vi "Begin.vi"(8 "error in":errorcluster) -> (0 "error out":errorcluster)   [LabVIEW 2018]
doc: "Called before other user functions, this VI is expected to open initial I/O refnums, load in file data, and do all program initialization. Notice that the <B>error out</B> terminal is simply used for data flow. Wiring it to other structures or subVIs ensures that this VI runs first."
uses:
  <vilib>/Rock Robotics/WPI/DriverStation/WPI_DriverStationRobotMode2.ctl
  <vilib>/Rock Robotics/WPI/Joystick/WPI_JoystickDeviceEnum.ctl
  <vilib>/Rock Robotics/SystemInterfaces/AI/FPGA_AIChannel.ctl
  <vilib>/Rock Robotics/WPI/Solenoid/WPI_SolenoidChannel.ctl
  <vilib>/Rock Robotics/SystemInterfaces/DIO/FPGA_DIORelayChannel.ctl
  <vilib>/Rock Robotics/WPI/Relay/WPI_RelayValue.ctl
  <vilib>/Rock Robotics/SystemInterfaces/DIO/FPGA_DIOPWMChannel.ctl
  <vilib>/Rock Robotics/SystemInterfaces/spilib/spi_bus.ctl
  <vilib>/Rock Robotics/SystemInterfaces/DIO/FPGA_DIOChannel.ctl
  Robot Global Data.vi
  <vilib>/Rock Robotics/WPI/Solenoid/WPI_SolenoidOpenSingle.vi
  <vilib>/Rock Robotics/WPI/Utilities/WPI_GetSetVariantRefNum.vi
  <vilib>/Rock Robotics/WPI/MotorControl/WPI_MotorControlOpen VictorSP.vi
  navx-mxp/labview/navX Library v2/IO/Open/Z900_navX_Open_SPI.vi
  <vilib>/Rock Robotics/WPI/Counter/WPI_CounterDigitalInputToDigitalSource.vi
  navx-mxp/labview/navX Library v2/navX Library v2.lvlib
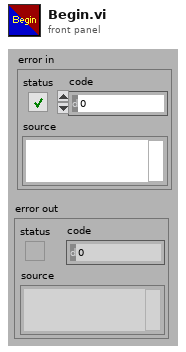
[diagram p1: front panel]
types:
  T1 = typedef "WPI_DriverStationRobotMode2.ctl" = enum16{"Autonomous Disabled", "Autonomous Enabled", "Teleop Disabled", "Teleop Enabled", "Disconnected", "Finish", "Test Disabled", "Test Enabled", "Emergency Stopped"}
  T2 = typedef "WPI_JoystickDeviceEnum.ctl" = enum16{"USB 0", "USB 1", "USB 2", "USB 3", "USB 4", "USB 5"}
  T3 = typedef "FPGA_AIChannel.ctl" = enum8{"AI 0", "AI 1", "AI 2", "AI 3", "AI MXP 0", "AI MXP 1", "AI MXP 2", "AI MXP 3", "Invalid"}
  T4 = typedef "FPGA_DIOPWMChannel.ctl" = enum8{"PWM 0", "PWM 1", "PWM 2", "PWM 3", "PWM 4", "PWM 5", "PWM 6", "PWM 7", "PWM 8", "PWM 9", "PWM MXP 0", "PWM MXP 1", "PWM MXP 2", "PWM MXP 3", "PWM MXP 4", "PWM MXP 5", "PWM MXP 6", "PWM MXP 7", "PWM MXP 8", "PWM MXP 9", "Invalid"}
  T5 = typedef "WPI_RelayValue.ctl" = enum16{"Off", "On", "Forward", "Reverse"}
  T6 = typedef "FPGA_DIORelayChannel.ctl" = enum8{"Relay 0", "Relay 1", "Relay 2", "Relay 3", "Invalid"}
  T7 = typedef "WPI_SolenoidChannel.ctl" = enum8{"Solenoid 0", "Solenoid 1", "Solenoid 2", "Solenoid 3", "Solenoid 4", "Solenoid 5", "Solenoid 6", "Solenoid 7", "Invalid"}
  T8 = typedef "spi_bus.ctl" = enum16{"SPI On-Board, CS0", "SPI On-Board, CS1", "SPI On-Board, CS2", "SPI On-Board, CS3", "SPI MXP", "Invalid"}
  T9 = typedef "WPI_JoystickDevRef.ctl" = cluster{"Device":T2}
  T10 = typedef "WPI_MotorControlDeviceRef.ctl" = cluster{"DeviceStatus":errorcluster, "Type":T11, "PWM":cluster{"PWM Channel":T4, "DeadBand":T12}, "CAN":cluster{"Device Number":u8, "SetOutput VI Ref":variant, "GetOutput VI Ref":variant, "Enable VI Ref":variant, "Disable VI Ref":variant, "Data":variant}, "Invert":bool, "DIO PWM":cluster{"PWM \"Enable\" Channel":T4, "DIOChannel":T13, "PWM Rate":dbl}}
  T11 = typedef "WPI_MotorControlType.ctl" = enum16{"PWM", "CAN", "DIO PWM"}
  T12 = typedef "WPI_PWMDeadband.ctl" = cluster{"Name":string, "maxPositivePwm":i32, "minPositivePwm":i32, "centerPwm":i32, "maxNegativePwm":i32, "minNegativePwm":i32, "angularRange":u16}
  T13 = typedef "FPGA_DIOChannel.ctl" = enum8{"DIO 0", "DIO 1", "DIO 2", "DIO 3", "DIO 4", "DIO 5", "DIO 6", "DIO 7", "DIO 8", "DIO 9", "DIO MXP 0", "DIO MXP 1", "DIO MXP 2", "DIO MXP 3", "DIO MXP 4", "DIO MXP 5", "DIO MXP 6", "DIO MXP 7", "DIO MXP 8", "DIO MXP 9", "DIO MXP 10", "DIO MXP 11", "DIO MXP 12", "DIO MXP 13", "DIO MXP 14", "DIO MXP 15", "SPI Port CS1", "SPI Port CS2", "SPI Port CS3", "SPI Port MISO", "SPI Port MOSI", "Invalid"}
  T14 = typedef "WPI_AnalogChannelDevRef.ctl" = cluster{"DevStatus":errorcluster, "Analog Channel":T3}
  T15 = typedef "WPI_CompressorDevRef.ctl" = cluster{"DevStatus":errorcluster, "Pneumatics Control Module":u8}
  T16 = typedef "WPI_RelayDevRef.ctl" = cluster{"DevStatus":errorcluster, "Relay Channel":T6, "Relay Direction":T17}
  T17 = typedef "WPI_RelayDirection.ctl" = enum16{"Both directions", "Forward only", "Reverse only"}
  T18 = typedef "WPI_SolenoidDevRef.ctl" = cluster{"DevStatus":errorcluster, "Pneumatics Control Module":u8, "Forward Solenoid Channel":T7, "Reverse Solenoid Channel":T7}
  T19 = typedef "navX Library v2.lvlib/Z900_navX_DeviceTypeDef.ctl" = cluster{"Interface":cluster{"Protocol":T20, "Update Rate (4Hz-100Hz)":u8, "navX Open TypeDef":variant}, "Notify Packet":refnum<notifier>, "Loop VI Refnum":refnum<vi>, "Ready to Close Occurrence Refnum":refnum<k4>}
  T20 = typedef "navX Library v2.lvlib/Z900_navX_ProtocolTypeDef.ctl" = enum16{"SERIAL", "I2C", "SPI"}
  T21 = typedef "WPI_DigitalInputDevRef.ctl" = cluster{"DevStatus":errorcluster, "DIO Channel":T13}
  T22 = typedef "FPGA_CounterEncoderSourceConvertionLVSourceType.ctl" = cluster{"DevStatus":errorcluster, "AnalogTriggerMode?":bool, "DigitalMode":cluster{"DIO Channel":T23}, "AnalogTriggerMode":cluster{"AnalogTriggerIndex":T24, "OutputType":T25}}
  T23 = typedef "FPGA_DIODigitalSourceChannel.ctl" = enum8{"DIO 0", "DIO 1", "DIO 2", "DIO 3", "DIO 4", "DIO 5", "DIO 6", "DIO 7", "DIO 8", "DIO 9", "DIO MXP 0", "DIO MXP 1", "DIO MXP 2", "DIO MXP 3", "DIO MXP 4", "DIO MXP 5", "DIO MXP 6", "DIO MXP 7", "DIO MXP 8", "DIO MXP 9", "DIO MXP 10", "DIO MXP 11", "DIO MXP 12", "DIO MXP 13", "DIO MXP 14", "DIO MXP 15", "SPI Port CS1", "SPI Port CS2", "SPI Port CS3", "SPI Port MISO", "SPI Port MOSI", "Disabled"}
  T24 = typedef "FPGA_AnalogTriggerIndex.ctl" = enum8{"Trig 0", "Trig 1", "Trig 2", "Trig 3", "Trig 4", "Trig 5", "Trig 6", "Trig 7", "Invalid"}
  T25 = typedef "FPGA_AnalogTriggerOutType.ctl" = enum16{"InWindow", "TriggerState", "Rising", "Falling"}
  T26 = typedef "WPI_EncoderDevRef.ctl" = cluster{"DevStatus":errorcluster, "EncoderIndex":T27, "CounterIndex":T28, "DistancePerCount":dbl, "Decoding Type":T29}
  T27 = typedef "FPGA_EncoderIdx.ctl" = enum8{"Enc 0", "Enc 1", "Enc 2", "Enc 3", "Enc 4", "Enc 5", "Enc 6", "Enc 7", "Invalid"}
  T28 = typedef "FPGA_CounterCtrSystemIndex.ctl" = enum8{"Ctr 0", "Ctr 1", "Ctr 2", "Ctr 3", "Ctr 4", "Ctr 5", "Ctr 6", "Ctr 7", "Invalid"}
  T29 = typedef "WPI_EncoderType.ctl" = enum16{"1x", "2x", "4x"}
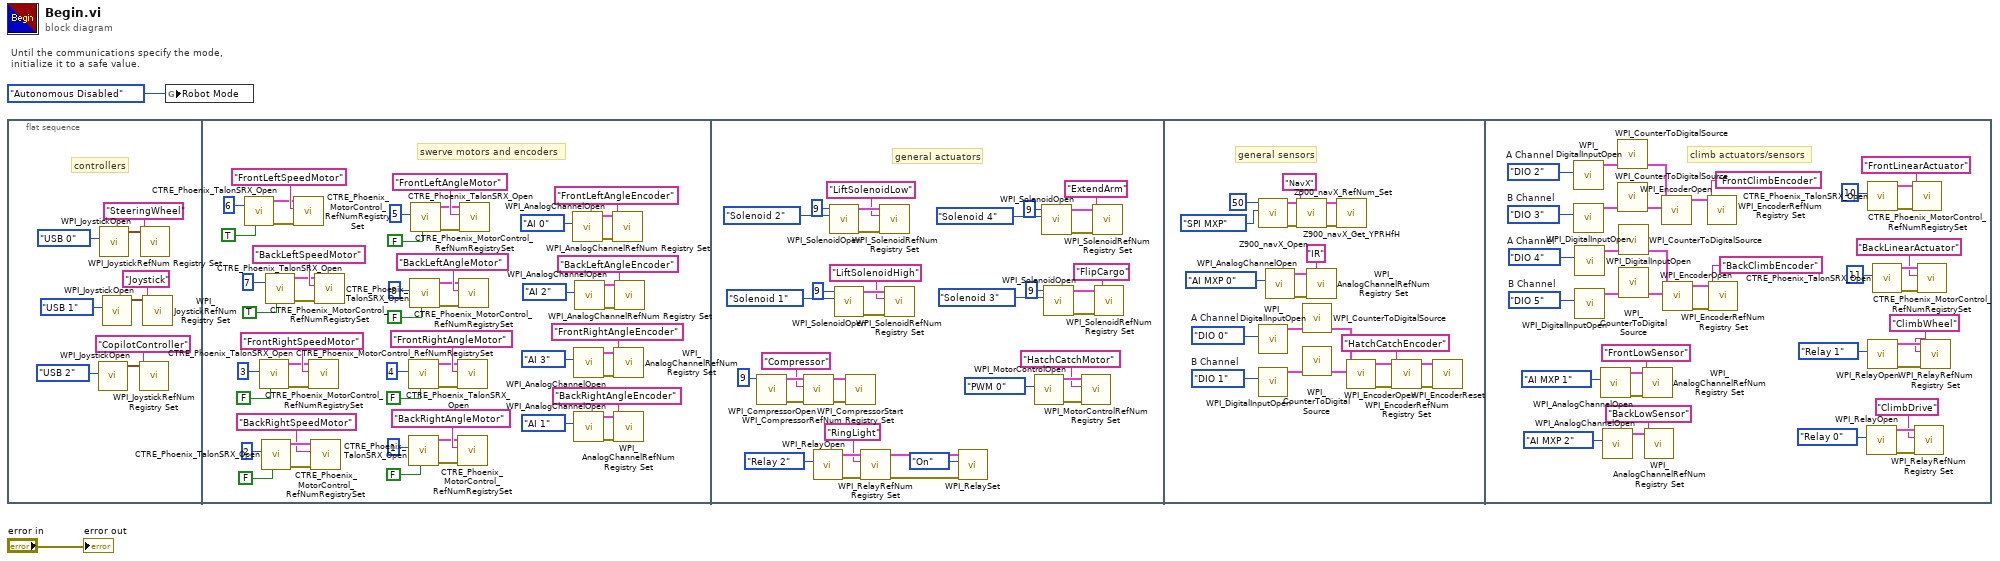
[diagram p0: block diagram]
diagram:
  # "Until the communications specify the mode,\ninitialize it to a safe value."
  n1 = flat-sequence {
    frame #0 {
      # "controllers"
      n2 = call <vilib>:"WPI_JoystickOpen.vi"("JoystickDevice"=WPI_JoystickDeviceEnum."USB 2") -> ("JoystickDevRef"=w5:T9)  [unwired: 10 in]
      n3 = call <vilib>:"WPI_JoystickOpen.vi"("JoystickDevice"=WPI_JoystickDeviceEnum."USB 0") -> ("JoystickDevRef"=w11:T9)  [unwired: 10 in]
      n4 = call <vilib>:"WPI_JoystickOpen.vi"("JoystickDevice"=WPI_JoystickDeviceEnum."USB 1") -> ("JoystickDevRef"=w8:T9)  [unwired: 10 in]
      n5 = call <vilib>:"WPI_JoystickRefNum Registry Set.vi"("refnum name"="CopilotController", "JoystickDevRef"=w5) -> ()  [unwired: 8 in, 2 out]
      n6 = call <vilib>:"WPI_JoystickRefNum Registry Set.vi"("refnum name"="SteeringWheel", "JoystickDevRef"=w11) -> ()  [unwired: 8 in, 2 out]
      n7 = call <vilib>:"WPI_JoystickRefNum Registry Set.vi"("refnum name"="Joystick", "JoystickDevRef"=w8) -> ()  [unwired: 8 in, 2 out]
    }
    frame #1 {
      # "swerve motors and encoders"
      n8 = call <vilib>:"CTRE_Phoenix_TalonSRX_Open.vi"("Invert"=TRUE, "Device Number"=u8 6) -> ("error out"=w53:errorcluster, "CAN Talon SRX Ref"=w54:T10)  [unwired: 8 in]
      n9 = call <vilib>:"CTRE_Phoenix_TalonSRX_Open.vi"("Invert"=FALSE, "Device Number"=u8 3) -> ("error out"=w57:errorcluster, "CAN Talon SRX Ref"=w58:T10)  [unwired: 8 in]
      n10 = call <vilib>:"CTRE_Phoenix_TalonSRX_Open.vi"("Invert"=FALSE, "Device Number"=u8 2) -> ("error out"=w59:errorcluster, "CAN Talon SRX Ref"=w60:T10)  [unwired: 8 in]
      n11 = call <vilib>:"CTRE_Phoenix_TalonSRX_Open.vi"("Invert"=TRUE, "Device Number"=u8 7) -> ("error out"=w55:errorcluster, "CAN Talon SRX Ref"=w56:T10)  [unwired: 8 in]
      n12 = call <vilib>:"CTRE_Phoenix_MotorControl_RefNumRegistrySet.vi"("error in (no error)"=w53, "refnum name"="FrontLeftSpeedMotor", "PhoenixMotorControlDevRef"=w54) -> ()  [unwired: 7 in, 2 out]
      n13 = call <vilib>:"CTRE_Phoenix_MotorControl_RefNumRegistrySet.vi"("error in (no error)"=w57, "refnum name"="FrontRightSpeedMotor", "PhoenixMotorControlDevRef"=w58) -> ()  [unwired: 7 in, 2 out]
      n14 = call <vilib>:"CTRE_Phoenix_MotorControl_RefNumRegistrySet.vi"("error in (no error)"=w59, "refnum name"="BackRightSpeedMotor", "PhoenixMotorControlDevRef"=w60) -> ()  [unwired: 7 in, 2 out]
      n15 = call <vilib>:"CTRE_Phoenix_MotorControl_RefNumRegistrySet.vi"("error in (no error)"=w55, "refnum name"="BackLeftSpeedMotor", "PhoenixMotorControlDevRef"=w56) -> ()  [unwired: 7 in, 2 out]
      n16 = call <vilib>:"CTRE_Phoenix_TalonSRX_Open.vi"("Invert"=FALSE, "Device Number"=u8 4) -> ("error out"=w39:errorcluster, "CAN Talon SRX Ref"=w40:T10)  [unwired: 8 in]
      n17 = call <vilib>:"CTRE_Phoenix_TalonSRX_Open.vi"("Invert"=FALSE, "Device Number"=u8 1) -> ("error out"=w37:errorcluster, "CAN Talon SRX Ref"=w38:T10)  [unwired: 8 in]
      n18 = call <vilib>:"CTRE_Phoenix_TalonSRX_Open.vi"("Invert"=FALSE, "Device Number"=u8 8) -> ("error out"=w41:errorcluster, "CAN Talon SRX Ref"=w42:T10)  [unwired: 8 in]
      n19 = call <vilib>:"CTRE_Phoenix_TalonSRX_Open.vi"("Invert"=FALSE, "Device Number"=u8 5) -> ("error out"=w43:errorcluster, "CAN Talon SRX Ref"=w44:T10)  [unwired: 8 in]
      n20 = call <vilib>:"CTRE_Phoenix_MotorControl_RefNumRegistrySet.vi"("error in (no error)"=w39, "refnum name"="FrontRightAngleMotor", "PhoenixMotorControlDevRef"=w40) -> ()  [unwired: 7 in, 2 out]
      n21 = call <vilib>:"CTRE_Phoenix_MotorControl_RefNumRegistrySet.vi"("error in (no error)"=w37, "refnum name"="BackRightAngleMotor", "PhoenixMotorControlDevRef"=w38) -> ()  [unwired: 7 in, 2 out]
      n22 = call <vilib>:"CTRE_Phoenix_MotorControl_RefNumRegistrySet.vi"("error in (no error)"=w41, "refnum name"="BackLeftAngleMotor", "PhoenixMotorControlDevRef"=w42) -> ()  [unwired: 7 in, 2 out]
      n23 = call <vilib>:"CTRE_Phoenix_MotorControl_RefNumRegistrySet.vi"("error in (no error)"=w43, "refnum name"="FrontLeftAngleMotor", "PhoenixMotorControlDevRef"=w44) -> ()  [unwired: 7 in, 2 out]
      n24 = call <vilib>:"WPI_AnalogChannelOpen.vi"("Analog Channel"=FPGA_AIChannel."AI 0") -> ("error out"=w35:errorcluster, "AIDeviceRef"=w36:T14)  [unwired: 9 in]
      n25 = call <vilib>:"WPI_AnalogChannelOpen.vi"("Analog Channel"=FPGA_AIChannel."AI 3") -> ("error out"=w27:errorcluster, "AIDeviceRef"=w28:T14)  [unwired: 9 in]
      n26 = call <vilib>:"WPI_AnalogChannelOpen.vi"("Analog Channel"=FPGA_AIChannel."AI 1") -> ("error out"=w23:errorcluster, "AIDeviceRef"=w24:T14)  [unwired: 9 in]
      n27 = call <vilib>:"WPI_AnalogChannelOpen.vi"("Analog Channel"=FPGA_AIChannel."AI 2") -> ("error out"=w31:errorcluster, "AIDeviceRef"=w32:T14)  [unwired: 9 in]
      n28 = call <vilib>:"WPI_AnalogChannelRefNum Registry Set.vi"("error in (no error)"=w35, "refnum name"="FrontLeftAngleEncoder", "AIDeviceRef"=w36) -> ()  [unwired: 7 in, 2 out]
      n29 = call <vilib>:"WPI_AnalogChannelRefNum Registry Set.vi"("error in (no error)"=w27, "refnum name"="FrontRightAngleEncoder", "AIDeviceRef"=w28) -> ()  [unwired: 7 in, 2 out]
      n30 = call <vilib>:"WPI_AnalogChannelRefNum Registry Set.vi"("error in (no error)"=w23, "refnum name"="BackRightAngleEncoder", "AIDeviceRef"=w24) -> ()  [unwired: 7 in, 2 out]
      n31 = call <vilib>:"WPI_AnalogChannelRefNum Registry Set.vi"("error in (no error)"=w31, "refnum name"="BackLeftAngleEncoder", "AIDeviceRef"=w32) -> ()  [unwired: 7 in, 2 out]
    }
    frame #2 {
      # "general actuators"
      n32 = call <vilib>:"WPI_CompressorOpen.vi"("Pneumatics Control Module (0)"=u8 9) -> ("CompressorDevRef"=w84:T15, "error out"=w83:errorcluster)  [unwired: 13 in]
      n33 = call <vilib>:"WPI_CompressorRefNum Registry Set.vi"("error in (no error)"=w83, "refnum name"="Compressor", "CompressorDevRef"=w84) -> ("error out"=w81:errorcluster, "CompressorDevRef"=w82:T15)  [unwired: 7 in]
      n34 = call <vilib>:"WPI_RelayOpen.vi"("Relay Channel"=FPGA_DIORelayChannel."Relay 2") -> ("error out"=w78:errorcluster, "RelayDevRef"=w77:T16)  [unwired: 9 in]
      n35 = call-poly <vilib>:"WPI_SolenoidOpen.vi"("Solenoid Channel"=WPI_SolenoidChannel."Solenoid 2", "Pneumatics Control Module (0)"=u8 9) -> ("error out"=w95:errorcluster, "SolenoidDevRef"=w104:T18)  [unwired: 8 in]
      n36 = call-poly <vilib>:"WPI_SolenoidOpen.vi"("Solenoid Channel"=WPI_SolenoidChannel."Solenoid 1", "Pneumatics Control Module (0)"=u8 9) -> ("error out"=w96:errorcluster, "SolenoidDevRef"=w102:T18)  [unwired: 8 in]
      n37 = call <vilib>:"WPI_CompressorStart.vi"("error in (no error)"=w81, "CompressorDevRef"=w82) -> ()  [unwired: 8 in, 2 out]
      n38 = call <vilib>:"WPI_RelayRefNum Registry Set.vi"("error in (no error)"=w78, "refnum name"="RingLight", "RelayDevRef"=w77) -> ("error out"=w75:errorcluster, "RelayDevRef"=w76:T16)  [unwired: 7 in]
      n39 = call <vilib>:"WPI_SolenoidRefNum Registry Set.vi"("error in (no error)"=w95, "refnum name"="LiftSolenoidLow", "SolenoidDevRef"=w104) -> ()  [unwired: 7 in, 2 out]
      n40 = call <vilib>:"WPI_SolenoidRefNum Registry Set.vi"("error in (no error)"=w96, "refnum name"="LiftSolenoidHigh", "SolenoidDevRef"=w102) -> ()  [unwired: 7 in, 2 out]
      n41 = call <vilib>:"WPI_RelaySet.vi"("error in (no error)"=w75, "RelayValue"=WPI_RelayValue."On", "RelayDevRef"=w76) -> ()  [unwired: 7 in, 2 out]
      n42 = call-poly <vilib>:"WPI_MotorControlOpen.vi"("PWM Channel"=FPGA_DIOPWMChannel."PWM 0") -> ("error out"=w71:errorcluster, "MotorControlDeviceRef"=w70:T10)  [unwired: 9 in]
      n43 = call-poly <vilib>:"WPI_SolenoidOpen.vi"("Solenoid Channel"=WPI_SolenoidChannel."Solenoid 4", "Pneumatics Control Module (0)"=u8 9) -> ("error out"=w90:errorcluster, "SolenoidDevRef"=w94:T18)  [unwired: 8 in]
      n44 = call-poly <vilib>:"WPI_SolenoidOpen.vi"("Solenoid Channel"=WPI_SolenoidChannel."Solenoid 3", "Pneumatics Control Module (0)"=u8 9) -> ("error out"=w85:errorcluster, "SolenoidDevRef"=w89:T18)  [unwired: 8 in]
      n45 = call <vilib>:"WPI_MotorControlRefNum Registry Set.vi"("error in (no error)"=w71, "refnum name"="HatchCatchMotor", "MotorControlDevRef"=w70) -> ()  [unwired: 7 in, 2 out]
      n46 = call <vilib>:"WPI_SolenoidRefNum Registry Set.vi"("error in (no error)"=w90, "refnum name"="ExtendArm", "SolenoidDevRef"=w94) -> ()  [unwired: 7 in, 2 out]
      n47 = call <vilib>:"WPI_SolenoidRefNum Registry Set.vi"("error in (no error)"=w85, "refnum name"="FlipCargo", "SolenoidDevRef"=w89) -> ()  [unwired: 7 in, 2 out]
    }
    frame #3 {
      w115 = FPGA_DIOChannel."DIO 1"  # B Channel
      w114 = FPGA_DIOChannel."DIO 0"  # A Channel
      # "general sensors"
      n48 = call-poly "Z900_navX_Open.vi"("SPI Bus"=spi_bus."SPI MXP", "Update Rate (4Hz-60Hz)"=u8 50) -> ("error out"=w126:errorcluster, "navX Device"=w125:T19)  [unwired: 8 in]
      n49 = call <vilib>:"WPI_DigitalInputOpen.vi"("DIO Channel"=w114) -> ("DigitalInputDevRef"=w111:T21)  [unwired: 1 in, 9 out]
      n50 = call <vilib>:"WPI_DigitalInputOpen.vi"("DIO Channel"=w115) -> ("DigitalInputDevRef"=w112:T21)  [unwired: 1 in, 9 out]
      n51 = call <vilib>:"WPI_AnalogChannelOpen.vi"("Analog Channel"=FPGA_AIChannel."AI MXP 0") -> ("error out"=w118:errorcluster, "AIDeviceRef"=w119:T14)  [unwired: 9 in]
      n52 = call "Z900_navX_RefNum_Set.vi"("error in (no error)"=w126, "refnum name"="NavX", "navX Device"=w125) -> ("error out"=w121:errorcluster, "navX Device"=w122:T19)  [unwired: 7 in]
      n53 = call-poly <vilib>:"WPI_CounterToDigitalSource.vi"("DigitalInputDevRef"=w111) -> ("Digital Source"=w110:T22)  [unwired: 6 out]
      n54 = call-poly <vilib>:"WPI_CounterToDigitalSource.vi"("DigitalInputDevRef"=w112) -> ("Digital Source"=w113:T22)  [unwired: 6 out]
      n55 = call <vilib>:"WPI_AnalogChannelRefNum Registry Set.vi"("error in (no error)"=w118, "refnum name"="IR", "AIDeviceRef"=w119) -> ()  [unwired: 7 in, 2 out]
      n56 = call "Z900_navX_Get_YPRHfH.vi"("error in (no error)"=w121, "navX Device"=w122) -> ()  [unwired: 6 in, 4 out]
      n57 = call <vilib>:"WPI_EncoderOpen.vi"("BSource"=w113, "ASource"=w110) -> ("error out"=w109:errorcluster, "EncoderDevRef"=w108:T26)  [unwired: 6 in, 2 out]
      n58 = call <vilib>:"WPI_EncoderRefNum Registry Set.vi"("error in (no error)"=w109, "refnum name"="HatchCatchEncoder", "EncoderDevRef"=w108) -> ("error out"=w106:errorcluster, "EncoderDevRef"=w105:T26)  [unwired: 7 in]
      n59 = call <vilib>:"WPI_EncoderReset.vi"("error in (no error)"=w106, "EncoderDevRef"=w105) -> ()  [unwired: 8 in, 2 out]
    }
    frame #4 {
      w151 = FPGA_DIOChannel."DIO 5"  # B Channel
      w150 = FPGA_DIOChannel."DIO 4"  # A Channel
      w160 = FPGA_DIOChannel."DIO 3"  # B Channel
      w159 = FPGA_DIOChannel."DIO 2"  # A Channel
      # "climb actuators/sensors"
      n60 = call <vilib>:"WPI_DigitalInputOpen.vi"("DIO Channel"=w159) -> ("DigitalInputDevRef"=w164:T21)  [unwired: 1 in, 9 out]
      n61 = call <vilib>:"WPI_DigitalInputOpen.vi"("DIO Channel"=w160) -> ("DigitalInputDevRef"=w165:T21)  [unwired: 1 in, 9 out]
      n62 = call <vilib>:"WPI_DigitalInputOpen.vi"("DIO Channel"=w150) -> ("DigitalInputDevRef"=w155:T21)  [unwired: 1 in, 9 out]
      n63 = call <vilib>:"WPI_DigitalInputOpen.vi"("DIO Channel"=w151) -> ("DigitalInputDevRef"=w154:T21)  [unwired: 1 in, 9 out]
      n64 = call <vilib>:"WPI_AnalogChannelOpen.vi"("Analog Channel"=FPGA_AIChannel."AI MXP 1") -> ("error out"=w136:errorcluster, "AIDeviceRef"=w137:T14)  [unwired: 9 in]
      n65 = call <vilib>:"WPI_AnalogChannelOpen.vi"("Analog Channel"=FPGA_AIChannel."AI MXP 2") -> ("AIDeviceRef"=w133:T14)  [unwired: 9 in, 1 out]
      n66 = call-poly <vilib>:"WPI_CounterToDigitalSource.vi"("DigitalInputDevRef"=w164) -> ("Digital Source"=w163:T22)  [unwired: 6 out]
      n67 = call-poly <vilib>:"WPI_CounterToDigitalSource.vi"("DigitalInputDevRef"=w165) -> ("Digital Source"=w166:T22)  [unwired: 6 out]
      n68 = call-poly <vilib>:"WPI_CounterToDigitalSource.vi"("DigitalInputDevRef"=w155) -> ("Digital Source"=w156:T22)  [unwired: 6 out]
      n69 = call-poly <vilib>:"WPI_CounterToDigitalSource.vi"("DigitalInputDevRef"=w154) -> ("Digital Source"=w153:T22)  [unwired: 6 out]
      n70 = call <vilib>:"WPI_AnalogChannelRefNum Registry Set.vi"("error in (no error)"=w136, "refnum name"="FrontLowSensor", "AIDeviceRef"=w137) -> ()  [unwired: 7 in, 2 out]
      n71 = call <vilib>:"WPI_AnalogChannelRefNum Registry Set.vi"("refnum name"="BackLowSensor", "AIDeviceRef"=w133) -> ()  [unwired: 8 in, 2 out]
      n72 = call <vilib>:"WPI_EncoderOpen.vi"("BSource"=w166, "ASource"=w163) -> ("EncoderDevRef"=w162:T26)  [unwired: 6 in, 3 out]
      n73 = call <vilib>:"WPI_EncoderOpen.vi"("BSource"=w153, "ASource"=w156) -> ("error out"=w157:errorcluster, "EncoderDevRef"=w158:T26)  [unwired: 6 in, 2 out]
      n74 = call <vilib>:"WPI_EncoderRefNum Registry Set.vi"("refnum name"="FrontClimbEncoder", "EncoderDevRef"=w162) -> ()  [unwired: 8 in, 2 out]
      n75 = call <vilib>:"WPI_EncoderRefNum Registry Set.vi"("error in (no error)"=w157, "refnum name"="BackClimbEncoder", "EncoderDevRef"=w158) -> ()  [unwired: 7 in, 2 out]
      n76 = call <vilib>:"WPI_RelayOpen.vi"("Relay Channel"=FPGA_DIORelayChannel."Relay 0") -> ("error out"=w141:errorcluster, "RelayDevRef"=w139:T16)  [unwired: 9 in]
      n77 = call <vilib>:"CTRE_Phoenix_TalonSRX_Open.vi"("Device Number"=u8 10) -> ("error out"=w149:errorcluster, "CAN Talon SRX Ref"=w148:T10)  [unwired: 9 in]
      n78 = call <vilib>:"WPI_RelayOpen.vi"("Relay Channel"=FPGA_DIORelayChannel."Relay 1") -> ("error out"=w130:errorcluster, "RelayDevRef"=w129:T16)  [unwired: 9 in]
      n79 = call <vilib>:"CTRE_Phoenix_TalonSRX_Open.vi"("Device Number"=u8 11) -> ("error out"=w145:errorcluster, "CAN Talon SRX Ref"=w144:T10)  [unwired: 9 in]
      n80 = call <vilib>:"CTRE_Phoenix_MotorControl_RefNumRegistrySet.vi"("error in (no error)"=w149, "refnum name"="FrontLinearActuator", "PhoenixMotorControlDevRef"=w148) -> ()  [unwired: 7 in, 2 out]
      n81 = call <vilib>:"WPI_RelayRefNum Registry Set.vi"("error in (no error)"=w141, "refnum name"="ClimbDrive", "RelayDevRef"=w139) -> ()  [unwired: 7 in, 2 out]
      n82 = call <vilib>:"CTRE_Phoenix_MotorControl_RefNumRegistrySet.vi"("error in (no error)"=w145, "refnum name"="BackLinearActuator", "PhoenixMotorControlDevRef"=w144) -> ()  [unwired: 7 in, 2 out]
      n83 = call <vilib>:"WPI_RelayRefNum Registry Set.vi"("error in (no error)"=w130, "refnum name"="ClimbWheel", "RelayDevRef"=w129) -> ()  [unwired: 7 in, 2 out]
    }
  }
  n84 = global write "Robot Global Data.vi" "Robot Mode"(WPI_DriverStationRobotMode2."Autonomous Disabled" ("Robot Mode")) -> ()
  "error out" <- "error in"
